vi "ConvertDataRateToTicks.vi"(1 "DataRate":u16) -> (0 "Ticks":u64)   [LabVIEW 2016, in "FPGAMockGyro.lvlib"]
uses:
  FPGAMockGyro.lvlib
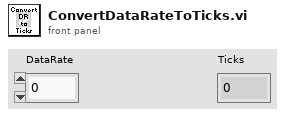
[diagram p1: front panel]
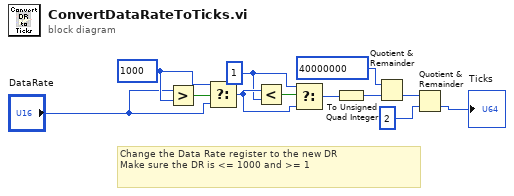
[diagram p0: block diagram]
diagram:
  w5 = u16 1 ("y")
  w4 = u16 1000 ("x")
  # "Change the Data Rate register to the new DR\nMake sure the DR is <= 1000 and >= 1"
  n1 = Greater?(x="DataRate", y=w4) -> (0:w3:bool)
  n2 = Select(t=w4, s=w3, f="DataRate") -> (s? t:f=w6:u16)
  n3 = Less?(x=w6, y=w5) -> (x < y?=w7:bool)
  n4 = Select(t=w5, s=w7, f=w6) -> (s? t:f=w11:u16)
  n5 = To Unsigned Quad Integer(1:w11) -> (0:w12:u64)
  n6 = Quotient & Remainder(x=u64 40000000, y=w12) -> (floor(x/y)=w9:u64)  [unwired: 1 out]
  n7 = Quotient & Remainder(x=w9, y=u64 2) -> (floor(x/y)=→"Ticks":u64)  [unwired: 1 out]
